vi "test folder list recrusive.vi"() -> ()   [LabVIEW 2023]
panel:
  out "size(s)":i32
  out "Array":path[](array[path])
  in  "path":path
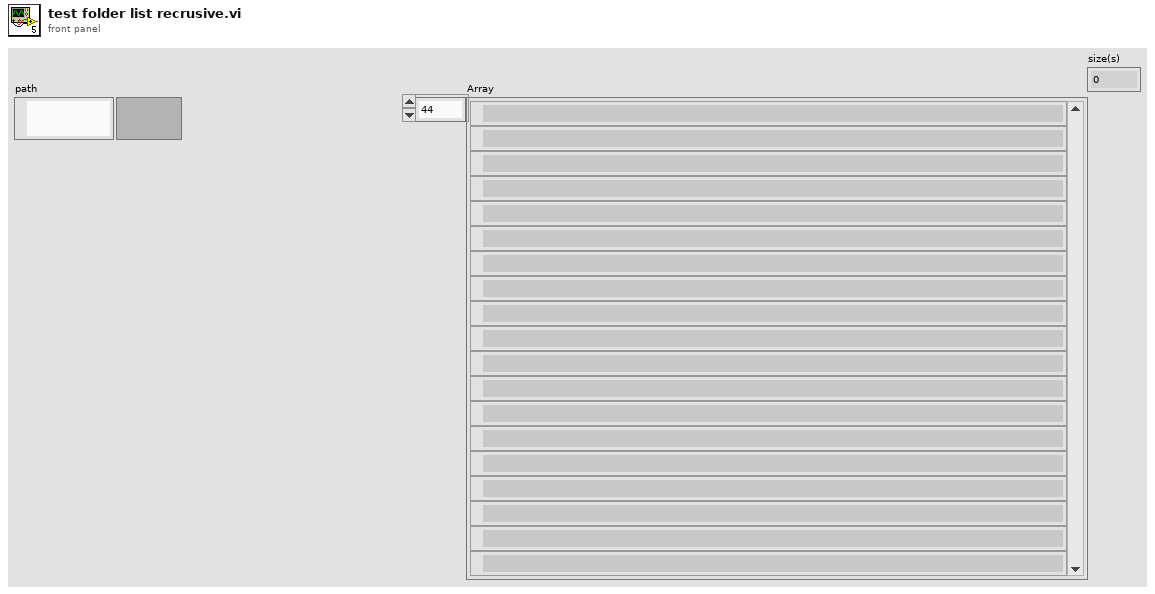
[diagram p1: front panel]
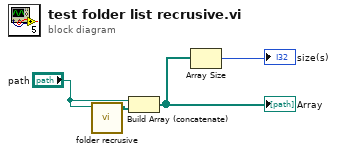
[diagram p0: block diagram]
diagram:
  n1 = call "folder recrusive.vi"("path"="path") -> ("Array"=w4:path[])  [unwired: 10 in]
  n2 = Build Array (concatenate)("path", w4) -> (w2:path[])
  "Array" <- w2
  n3 = Array Size(array=w2) -> (size(s)=→"size(s)":i32)
